vi "개별읽기응답(SubVI).vi"(1 "응답 프레임":string) -> (0 "Word 배열(U16)":u16[](array[numeric]) format="%.0x")   [LabVIEW 2014]
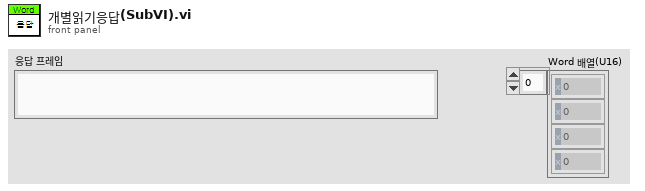
[diagram p1: front panel]
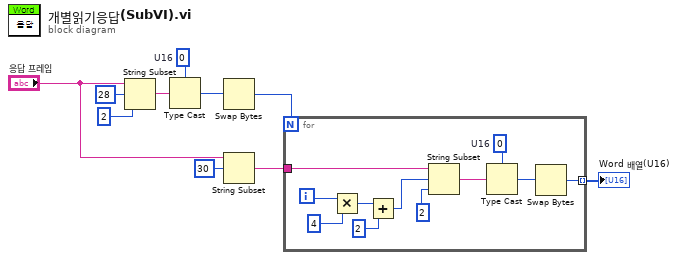
[diagram p0: block diagram]
diagram:
  w3 = u16 0  # U16
  n1 = String Subset(string="응답 프레임", offset (0)=28 ("오프셋(0)"), length (rest)=2 ("길이(나머지)")) -> (substring=w4:string)
  n2 = Type Cast(type=w3, x=w4) -> (*(type *) &x=w2:u16)
  n3 = Swap Bytes(anything=w2) -> (byte swapped=w1:u16)
  n4 = String Subset(string="응답 프레임", offset (0)=30 ("오프셋(0)")) -> (substring=w6:string)  [unwired: 1 in]
  n5 = for {
    N: w1 -> [_]
    tunnel: w6 -> [w17]
    tunnel: [w11] -> w5 mode=indexing
    i -> [w21]
    w13 = u16 0  # U16
    n6 = Multiply(x=w21, y=4) -> (x*y=w19:i32)
    n7 = Add(x=w19, y=2 ("x")) -> (x+y=w16:i32)
    n8 = String Subset(string=w17, offset (0)=w16, length (rest)=2 ("길이(나머지)")) -> (substring=w12:string)
    n9 = Type Cast(type=w13, x=w12) -> (*(type *) &x=w14:u16)
    n10 = Swap Bytes(anything=w14) -> (byte swapped=w11:u16)
  }
  "Word 배열(U16)" <- w5
